vi "Set Chan Default for typedefs.vi"(8 "error in":errorcluster, 10 "Ctl Ref":refnum<vi>, 11 "Section Ref in":T1 format="%.0x") -> (0 "error out":errorcluster, 3 "Section Ref out":T1 format="%.0x")   [LabVIEW 2016, in "DCM System Explorer.lvlib"]
uses:
  DCM System Explorer.lvlib
  <vilib>/NI Veristand/Custom Device API/Custom Device Item Ref.ctl
  <vilib>/NI VeriStand/Custom Device API/Custom Device API.lvlib
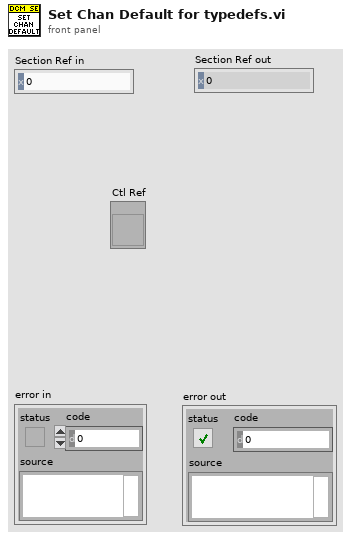
[diagram p1: front panel]
types:
  T1 = typedef "Custom Device API.lvlib/Custom Device Item Ref.ctl" = u64
  T2 = cluster{"Index Ref":refnum<vi>, "Array Refs":refnum<vi>[], "Array Positions":i32[][], "Device Ref":T1, "Section Ref":T1, "GUIDChDelProt":string, "GUIDSectDelProt":string}
  T3 = cluster{"Index Ref":refnum<vi>, "Array Refs":refnum<vi>[], "Array Positions":i32[][], "Device Ref":T1, "Section Ref":T1, "GUIDChDelProt":string, "GUIDSectDelProt":string}[]
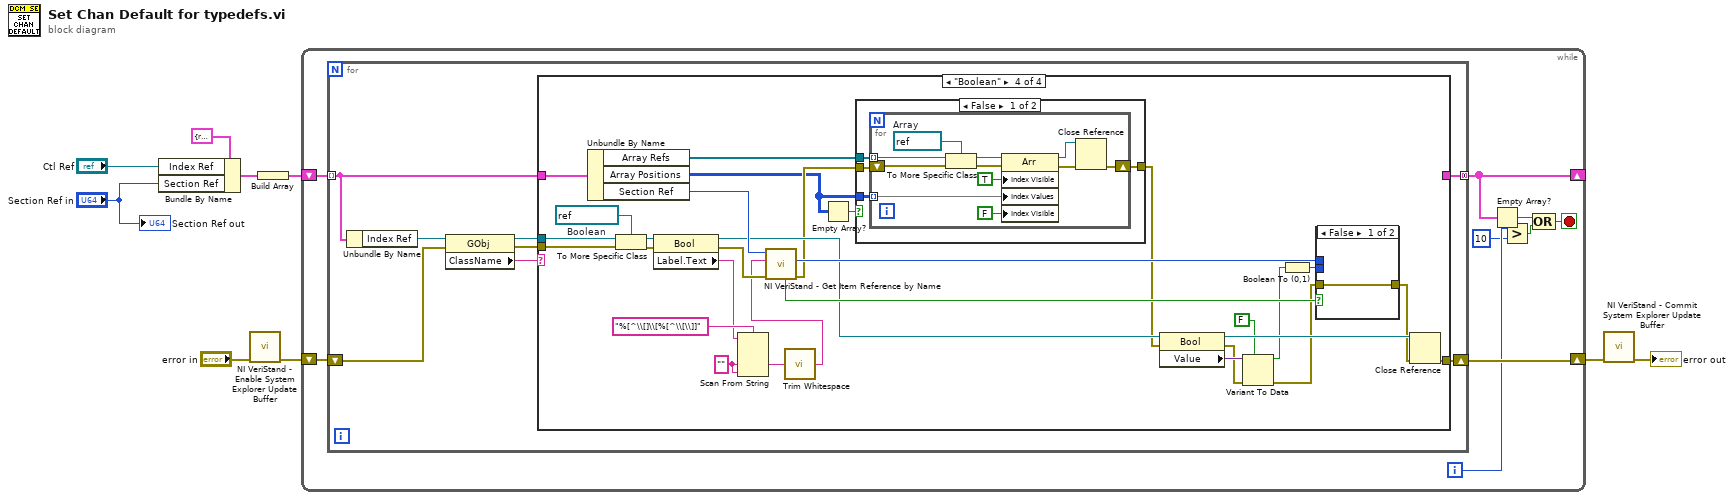
[diagram p0: block diagram]
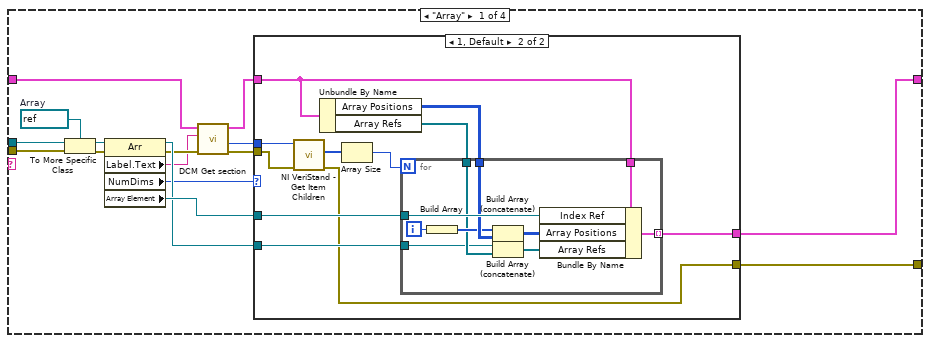
[diagram p2: hidden frame]
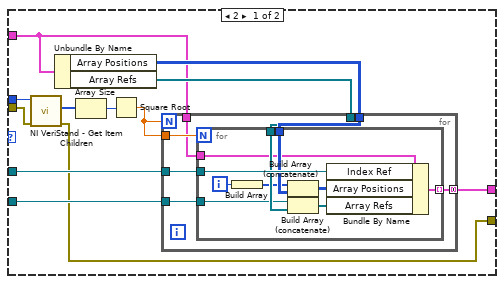
[diagram p3: hidden frame]
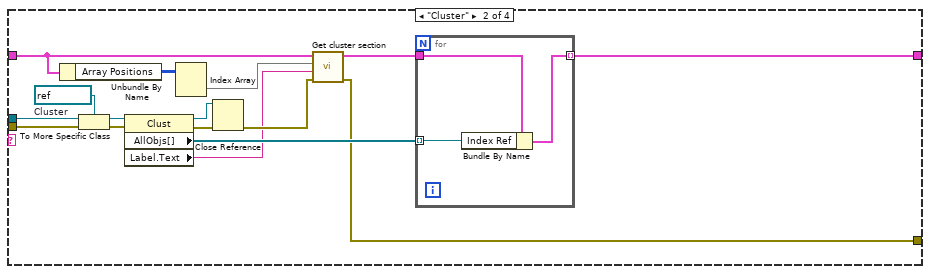
[diagram p4: hidden frame]
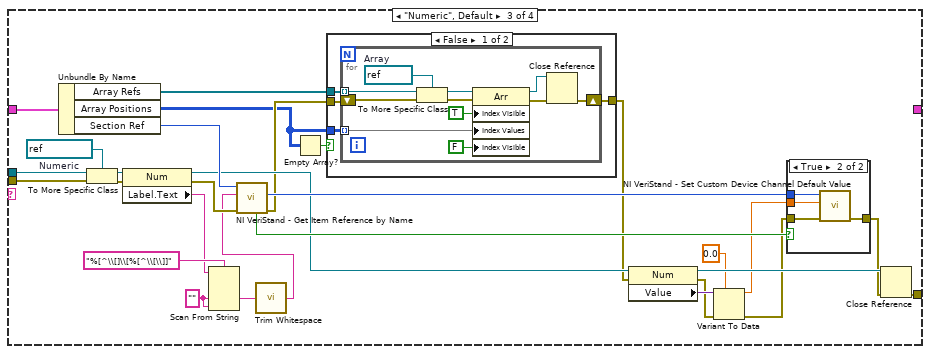
[diagram p5: hidden frame]
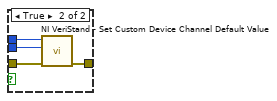
[diagram p8: hidden frame]
diagram:
  n1 = Bundle By Name(cluster=T2 {"Index Ref"=refnum, "Array Refs"=[], "Array Positions"=[], "Device Ref"=0, "Section Ref"=0, "GUIDChDelProt"="", "GUIDSectDelProt"=""} ("Data"), "Index Ref"="Ctl Ref", "Section Ref"="Section Ref in") -> (w8:T2)
  n2 = call <vilib>:"NI VeriStand - Enable System Explorer Update Buffer.vi"("error in (no error)"="error in") -> ("error out"=w3:errorcluster)  [unwired: 10 in]
  n3 = Build Array(w8) -> (w9:T3)
  n4 = while {
    shift-right: [w17] -> _
    shift-left: w9 -> [w18]
    shift-right: [w16] -> w2
    shift-left: w3 -> [w15]
    i -> [w12]
    stop <- w13 stop-if-true
    n5 = for {
      tunnel: w18 -> [w23] mode=indexing
      tunnel: [w19] -> w17 mode=concatenating
      shift-right: [w24] -> w16
      shift-left: w15 -> [w20]
      n6 = Unbundle By Name(w23) -> ("Index Ref"=w25:refnum<vi>)
      n7 = property class="GObj"(reference=w25, error in=w20) -> (reference out=w26:refnum<vi>, error out=w21:errorcluster, "ClassName"=w22:string)
      n8 = case shown="\"Boolean\"" w22 {
        tunnel: w26 -> [w42 w106 w140 w191]
        tunnel: w21 -> [w39 w105 w138 w189]
        tunnel: [w36 w94 w132 w183] -> w24
        tunnel: w23 -> [w34 w98 w137 w188]
        tunnel: [w37 w99 _ _] -> w19
        frame "Array" {
          w38 = refnum<vi> refnum  # Array
          n9 = To More Specific Class(target class=w38, reference=w42, error in=w39) -> (specific class reference=w41:refnum<vi>, error out=w40:errorcluster)
          n10 = property class="Arr"(reference=w41, error in=w40) -> (reference out=w31:refnum<vi>, error out=w30:errorcluster, "Label.Text"=w27:string, "NumDims"=w28:u32, "Array Element"=w35:refnum<vi>)
          n11 = call "DCM Get section.vi"("error in"=w30, "Label.Text in"=w27, "Data in"=w34) -> ("error out"=w32:errorcluster, "Section Ptr"=w29:T1, "Data out"=w33:T2)  [unwired: 6 in]
          n12 = case shown="1, Default" w28 {
            tunnel: w32 -> [w47 w72]
            tunnel: w33 -> [w50 w78]
            tunnel: [w54 w82] -> w37
            tunnel: [w45 w75] -> w36
            tunnel: w35 -> [w53 w81]
            tunnel: w31 -> [w49 w77]
            tunnel: w29 -> [w48 w73]
            frame 2 {
              n13 = call <vilib>:"NI VeriStand - Get Item Children.vi"("error in (no error)"=w47, "Item Ref in"=w48) -> ("error out"=w45:errorcluster, "Child Refs"=w46:T1[])  [unwired: 6 in, 2 out]
              n14 = Unbundle By Name(w50) -> ("Array Positions"=w52:i32[][], "Array Refs"=w51:refnum<vi>[])
              n15 = Array Size(array=w46) -> (size(s)=w44:i32)
              n16 = Square Root(x=w44) -> (sqrt(x)=w43:dbl)
              n17 = for {
                N: w43 -> [_]
                tunnel: w43 -> [w61]
                tunnel: [w59] -> w54 mode=concatenating
                tunnel: w53 -> [w60]
                tunnel: w49 -> [w58]
                tunnel: w52 -> [w57]
                tunnel: w51 -> [w56]
                tunnel: w50 -> [w55]
                n18 = for {
                  N: w61 -> [_]
                  tunnel: w60 -> [w69]
                  tunnel: [w70] -> w59 mode=indexing
                  tunnel: w58 -> [w65]
                  tunnel: w57 -> [w64]
                  tunnel: w56 -> [w66]
                  tunnel: w55 -> [w62]
                  i -> [w71]
                  n19 = Build Array(w71) -> (w63:i32[])
                  n20 = Build Array (concatenate)(w63, w64) -> (w68:i32[][])
                  n21 = Build Array (concatenate)(w65, w66) -> (w67:refnum<vi>[])
                  n22 = Bundle By Name(cluster=w62, "Index Ref"=w69, "Array Positions"=w68, "Array Refs"=w67) -> (w70:T2)
                }
              }
            }
            frame 1, Default {
              n23 = call <vilib>:"NI VeriStand - Get Item Children.vi"("error in (no error)"=w72, "Item Ref in"=w73) -> ("error out"=w75:errorcluster, "Child Refs"=w76:T1[])  [unwired: 6 in, 2 out]
              n24 = Unbundle By Name(w78) -> ("Array Positions"=w80:i32[][], "Array Refs"=w79:refnum<vi>[])
              n25 = Array Size(array=w76) -> (size(s)=w74:i32)
              n26 = for {
                N: w74 -> [_]
                tunnel: w78 -> [w92]
                tunnel: [w91] -> w82 mode=indexing
                tunnel: w81 -> [w89]
                tunnel: w77 -> [w83]
                tunnel: w80 -> [w86]
                tunnel: w79 -> [w84]
                i -> [w90]
                n27 = Build Array(w90) -> (w85:i32[])
                n28 = Build Array (concatenate)(w85, w86) -> (w88:i32[][])
                n29 = Build Array (concatenate)(w83, w84) -> (w87:refnum<vi>[])
                n30 = Bundle By Name(cluster=w92, "Index Ref"=w89, "Array Positions"=w88, "Array Refs"=w87) -> (w91:T2)
              }
            }
          }
        }
        frame "Cluster" {
          w104 = refnum<vi> refnum  # Cluster
          n31 = Unbundle By Name(w98) -> ("Array Positions"=w102:i32[][])
          n32 = To More Specific Class(target class=w104, reference=w106, error in=w105) -> (specific class reference=w108:refnum<vi>, error out=w107:errorcluster)
          n33 = property class="Clust"(reference=w108, error in=w107) -> (reference out=w101:refnum<vi>, error out=w100:errorcluster, "AllObjs[]"=w103:refnum<vi>[], "Label.Text"=w93:string)
          n34 = Index Array(array=w102) -> (element=w97:i32[])  [unwired: 2 in]
          n35 = Close Reference(reference=w101, error in (no error)=w100) -> (error out=w95:errorcluster)
          n36 = call "Get cluster section.vi"("error in (no error)"=w95, "Name (none)"=w93, "Array Positions (none)"=w97, "Data in"=w98) -> ("error out"=w94:errorcluster, "Data out"=w96:T2)  [unwired: 4 in, 2 out]
          n37 = for {
            tunnel: w96 -> [w110]
            tunnel: w103 -> [w109] mode=indexing
            tunnel: [w111] -> w99 mode=indexing
            n38 = Bundle By Name(cluster=w110, "Index Ref"=w109) -> (w111:T2)
          }
        }
        frame "Numeric", Default {
          w131 = "" ("default value 2")
          w136 = refnum<vi> refnum  # Numeric
          n39 = Unbundle By Name(w137) -> ("Array Refs"=w134:refnum<vi>[], "Array Positions"=w112:i32[][], "Section Ref"=w128:T1)
          n40 = To More Specific Class(target class=w136, reference=w140, error in=w138) -> (specific class reference=w139:refnum<vi>, error out=w135:errorcluster)
          n41 = property class="Num"(reference=w139, error in=w135) -> (reference out=w124:refnum<vi>, error out=w127:errorcluster, "Label.Text"=w123:string)
          n42 = Scan From String(format string="%[^\\[]\\[%[^\\[\\]]" ("regular expression"), input string=w123, default 1=w131, default 2=w131) -> (output 1=w130:string)  [unwired: 3 in, 3 out]
          n43 = call <vilib>:"Trim Whitespace.vi"("string"=w130) -> ("trimmed string"=w114:string)  [unwired: 1 in]
          n44 = call <vilib>:"NI VeriStand - Get Item Reference by Name.vi"("error in (no error)"=w127, "Item Name"=w114, "Parent Ref in"=w128) -> ("error out"=w122:errorcluster, "Item Ref"=w126:T1, "Found"=w125:bool)  [unwired: 5 in, 1 out]
          n45 = Empty Array?(array=w112) -> (empty?=w113:bool)
          n46 = case shown="False" w113 {
            tunnel: w134 -> [w149 _]
            tunnel: w112 -> [w148 _]
            tunnel: w122 -> [w146 w161]
            tunnel: [w147 w161] -> w118
            frame False {
              n47 = for {
                tunnel: w149 -> [w154] mode=indexing
                tunnel: w148 -> [w158] mode=indexing
                shift-right: [w151] -> w147
                shift-left: w146 -> [w156]
                w160 = refnum<vi> refnum  # Array
                n48 = To More Specific Class(target class=w160, reference=w154, error in=w156) -> (specific class reference=w159:refnum<vi>, error out=w155:errorcluster)
                n49 = property class="Arr"(reference=w159, error in=w155, "Index Visible"=TRUE, "Index Values"=w158, "Index Visible"=FALSE) -> (reference out=w152:refnum<vi>, error out=w153:errorcluster)
                n50 = Close Reference(reference=w152, error in (no error)=w153) -> (error out=w151:errorcluster)
              }
            }
            frame True {
            }
          }
          n51 = property class="Num"(reference=w124, error in=w118) -> (reference out=w133:refnum<vi>, error out=w119:errorcluster, "Value"=w121:variant)
          n52 = Variant To Data(error in=w119, type=0.0, Variant=w121) -> (data=w116:dbl, error out=w117:errorcluster)
          n53 = case shown="True" w125 {
            tunnel: [w141 w145] -> w115
            tunnel: w117 -> [w141 w144]
            tunnel: w126 -> [_ w143]
            tunnel: w116 -> [_ w142]
            frame False {
            }
            frame True {
              n54 = call <vilib>:"NI VeriStand - Set Custom Device Channel Default Value.vi"("error in (no error)"=w144, "Default Value"=w142, "Channel Ref in"=w143) -> ("error out"=w145:errorcluster)  [unwired: 7 in, 1 out]
            }
          }
          n55 = Close Reference(reference=w133, error in (no error)=w115) -> (error out=w132:errorcluster)
        }
        frame "Boolean" {
          w182 = "" ("default value 2")
          w187 = refnum<vi> refnum  # Boolean
          n56 = Unbundle By Name(w188) -> ("Array Refs"=w185:refnum<vi>[], "Array Positions"=w162:i32[][], "Section Ref"=w179:T1)
          n57 = To More Specific Class(target class=w187, reference=w191, error in=w189) -> (specific class reference=w190:refnum<vi>, error out=w186:errorcluster)
          n58 = property class="Bool"(reference=w190, error in=w186) -> (reference out=w175:refnum<vi>, error out=w178:errorcluster, "Label.Text"=w174:string)
          n59 = Scan From String(format string="%[^\\[]\\[%[^\\[\\]]" ("regular expression"), input string=w174, default 1=w182, default 2=w182) -> (output 1=w181:string)  [unwired: 3 in, 3 out]
          n60 = call <vilib>:"Trim Whitespace.vi"("string"=w181) -> ("trimmed string"=w164:string)  [unwired: 1 in]
          n61 = call <vilib>:"NI VeriStand - Get Item Reference by Name.vi"("error in (no error)"=w178, "Item Name"=w164, "Parent Ref in"=w179) -> ("error out"=w173:errorcluster, "Item Ref"=w177:T1, "Found"=w176:bool)  [unwired: 5 in, 1 out]
          n62 = Empty Array?(array=w162) -> (empty?=w163:bool)
          n63 = case shown="False" w163 {
            tunnel: w185 -> [w200 _]
            tunnel: w162 -> [w199 _]
            tunnel: w173 -> [w197 w212]
            tunnel: [w198 w212] -> w170
            frame False {
              n64 = for {
                tunnel: w200 -> [w205] mode=indexing
                tunnel: w199 -> [w209] mode=indexing
                shift-right: [w202] -> w198
                shift-left: w197 -> [w207]
                w211 = refnum<vi> refnum  # Array
                n65 = To More Specific Class(target class=w211, reference=w205, error in=w207) -> (specific class reference=w210:refnum<vi>, error out=w206:errorcluster)
                n66 = property class="Arr"(reference=w210, error in=w206, "Index Visible"=TRUE, "Index Values"=w209, "Index Visible"=FALSE) -> (reference out=w203:refnum<vi>, error out=w204:errorcluster)
                n67 = Close Reference(reference=w203, error in (no error)=w204) -> (error out=w202:errorcluster)
              }
            }
            frame True {
            }
          }
          n68 = property class="Bool"(reference=w175, error in=w170) -> (reference out=w184:refnum<vi>, error out=w171:errorcluster, "Value"=w172:variant)
          n69 = Variant To Data(error in=w171, type=FALSE, Variant=w172) -> (data=w165:bool, error out=w169:errorcluster)
          n70 = Boolean To (0,1)(Boolean=w165) -> (0, 1=w166:i16)
          n71 = case shown="False" w176 {
            tunnel: [w192 w196] -> w168
            tunnel: w169 -> [w192 w195]
            tunnel: w177 -> [_ w194]
            tunnel: w166 -> [_ w193]
            frame False {
            }
            frame True {
              n72 = call <vilib>:"NI VeriStand - Set Custom Device Channel Default Value.vi"("error in (no error)"=w195, "Default Value"=w193, "Channel Ref in"=w194) -> ("error out"=w196:errorcluster)  [unwired: 7 in, 1 out]
            }
          }
          n73 = Close Reference(reference=w184, error in (no error)=w168) -> (error out=w183:errorcluster)
        }
      }
    }
    n74 = Empty Array?(array=w17) -> (empty?=w14:bool)
    n75 = Greater?(x=w12, y=10) -> (0:w10:bool)
    n76 = Compound Arithmetic op=OR(w14, w10) -> (w13:bool)
  }
  n77 = call <vilib>:"NI VeriStand - Commit System Explorer Update Buffer.vi"("error in (no error)"=w2) -> ("error out"=→"error out":errorcluster)  [unwired: 10 in]
  "Section Ref out" <- "Section Ref in"
